vi "Pump Init Selection.vi"(8 "error in (no error)":errorcluster, 11 "Pump Settings In":T1 {"Masterflex"."Pump Number" min=1.0 max=20.0 step=1.0; "Ismatech"."Pump Number" min=1.0 max=20.0 step=1.0; "ASIA Pump C"."channel" min=-1 max=1 step=1}) -> (0 "error out":errorcluster, 2 "Initialized":bool, 3 "Pump Settings Out":T1 {"Masterflex"."Pump Number" min=1.0 max=20.0 step=1.0; "Ismatech"."Pump Number" min=1.0 max=20.0 step=1.0; "ASIA Pump C"."channel" min=-1 max=1 step=1})   [LabVIEW 2018, in "Pump Module.lvlib" / "Pump Module Engine.lvlib"]
uses:
  Pump Module Engine.lvlib
  Pump Settings Cluster.ctl
  Measure Instrument/PID 2 Output Enum.ctl
  Masterflex 7550-30/Controls/Settings Cluster.ctl
  Ismatec ISM 831C/Controls/Ismatech Settings Cluster.ctl
  VICI M50 Party Mode/Settings Cluster.ctl
  Tacmina QI/Tacmina QI DAQ Setting.ctl
  KNF Pump/Settings Cluster plus SIMDOS.ctl
  ASIA Pump/Pump Settings.ctl
  FLOM Pump/Settings Cluster.ctl
  SSI PR Class/SSI PR Settings Cluster.ctl
  Masterflex 75211/Masterflex 75211 DAQ Setting.ctl
  Ismatec ISM 831C/Ismatec ISM 831C.lvlib
  Masterflex 7550-30/Masterflex 7550-30.lvlib
  VICI M50 Party Mode/VICI M6 M50 Party Mode.lvlib
  Tacmina QI/Tacmina QI.lvlib
  KNF Pump/KNF SIMDOS.lvlib
  ASIA Pump.lvlib
  FLOM Pump/FLOM Pump.lvlib
  SSI PR Class/SSI PR Pump.lvlib
  Masterflex 75211/Masterflex 75211.lvlib
  Pump Module.lvlib
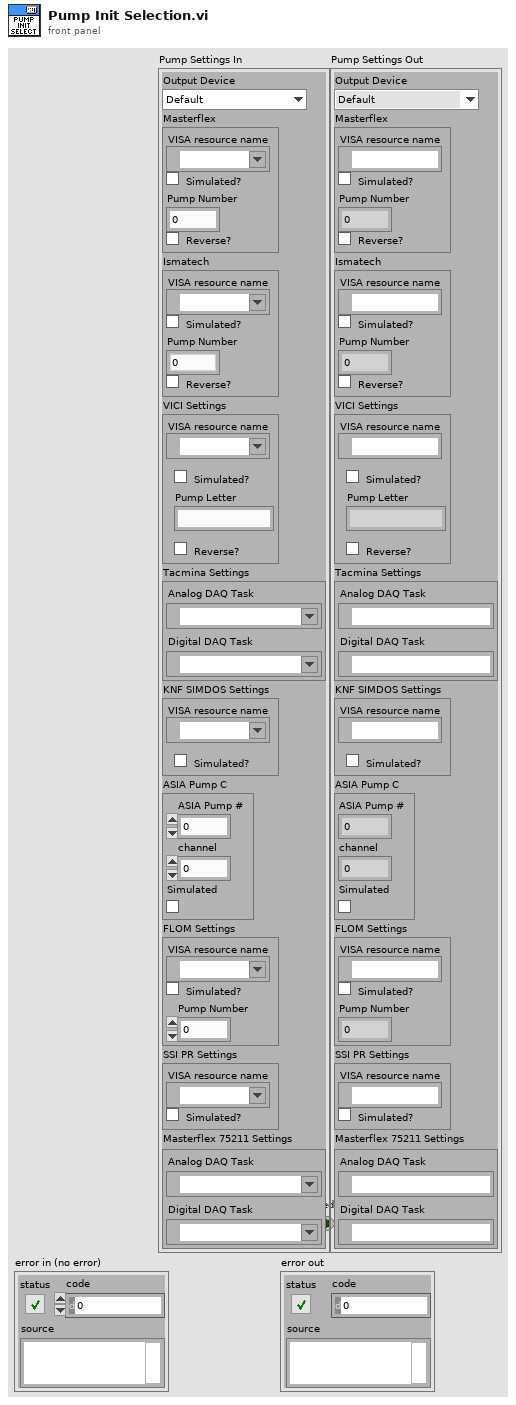
[diagram p1: front panel]
types:
  T1 = typedef "Pump Module.lvlib/Pump Settings Cluster.ctl" = cluster{"Output Device":T2, "Masterflex":T3, "Ismatech":T4, "VICI Settings":T5, "Tacmina Settings":T6, "KNF SIMDOS Settings":T7, "ASIA Pump C":T8, "FLOM Settings":T9, "SSI PR Settings":T10, "Masterflex 75211 Settings":T11}
  T2 = typedef "PID 2 Output Enum.ctl" = enum16{"Default", "Ismatec ISM 831C", "Masterflex 7550-30", "VICI", "Tacmina QI", "KNF SIMDOS", "ASIA Type C", "FLOM UI-22-11", "SSI PR", "Masterflex 75211-70"}
  T3 = typedef "Masterflex 7550-30.lvlib/Settings Cluster.ctl" = cluster{"VISA resource name":refnum<visa-resource-name>, "Simulated?":bool, "Pump Number":dbl, "Reverse?":bool}
  T4 = typedef "Ismatec ISM 831C.lvlib/Ismatech Settings Cluster.ctl" = cluster{"VISA resource name":refnum<visa-resource-name>, "Simulated?":bool, "Pump Number":dbl, "Reverse?":bool}
  T5 = typedef "VICI M6 M50 Party Mode.lvlib/Settings Cluster.ctl" = cluster{"VISA resource name":refnum<visa-resource-name>, "Simulated?":bool, "Pump Letter":string, "Reverse?":bool}
  T6 = typedef "Tacmina QI.lvlib/Tacmina QI DAQ Setting.ctl" = cluster{"Analog DAQ Task":refnum<k21>, "Digital DAQ Task":refnum<k21>}
  T7 = typedef "KNF SIMDOS.lvlib/Settings Cluster plus SIMDOS.ctl" = cluster{"VISA resource name":refnum<visa-resource-name>, "Simulated?":bool}
  T8 = typedef "ASIA Pump.lvlib/Pump Settings.ctl" = cluster{"ASIA Pump #":i32, "channel":i32, "Simulated":bool}
  T9 = typedef "FLOM Pump.lvlib/Settings Cluster.ctl" = cluster{"VISA resource name":refnum<visa-resource-name>, "Simulated?":bool, "Pump Number":dbl}
  T10 = typedef "SSI PR Pump.lvlib/SSI PR Settings Cluster.ctl" = cluster{"VISA resource name":refnum<visa-resource-name>, "Simulated?":bool}
  T11 = typedef "Masterflex 75211.lvlib/Masterflex 75211 DAQ Setting.ctl" = cluster{"Analog DAQ Task":refnum<k21>, "Digital DAQ Task":refnum<k21>}
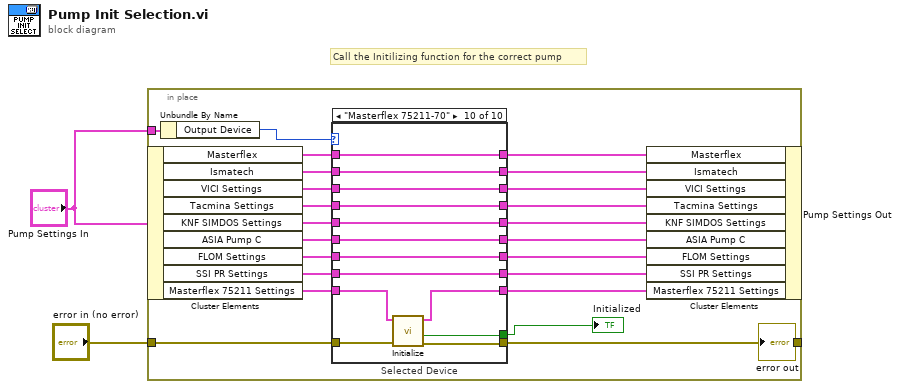
[diagram p0: block diagram]
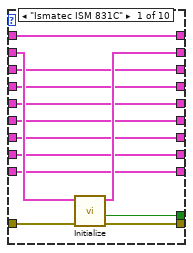
[diagram p2: hidden frame]
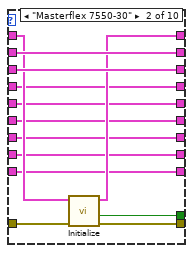
[diagram p3: hidden frame]
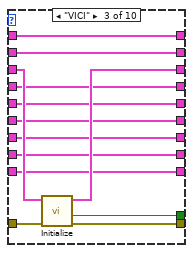
[diagram p4: hidden frame]
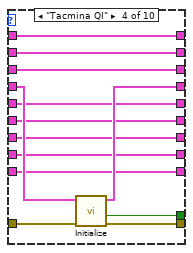
[diagram p5: hidden frame]
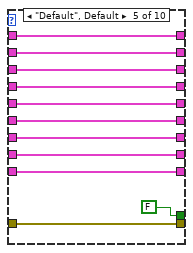
[diagram p6: hidden frame]
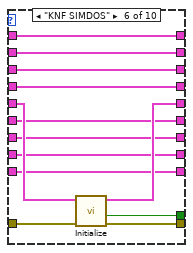
[diagram p7: hidden frame]
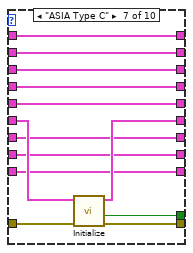
[diagram p8: hidden frame]
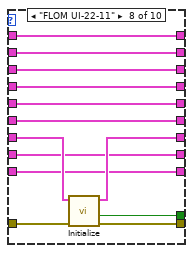
[diagram p9: hidden frame]
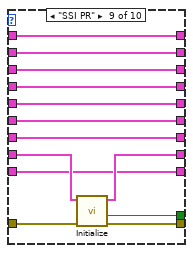
[diagram p10: hidden frame]
diagram:
  # "Call the Initilizing function for the correct pump"
  n1 = in-place {
    in-place-border: [w25] -> w4
    in-place-border: "error in (no error)" -> [w24]
    in-place-border: "Pump Settings In" -> [w23]
    n2 = in-place-cluster #1("Pump Settings In") -> ("Masterflex"=w22:T3, "Ismatech"=w21:T4, "VICI Settings"=w20:T5, "Tacmina Settings"=w19:T6, "KNF SIMDOS Settings"=w18:T7, "ASIA Pump C"=w17:T8, "FLOM Settings"=w16:T9, "SSI PR Settings"=w15:T10, "Masterflex 75211 Settings"=w5:T11)
    n3 = Unbundle By Name(w23) -> ("Output Device"=w26:T2)
    n4 = case "Selected Device" shown="\"Masterflex 75211-70\"" w26 {
      tunnel: w22 -> [w37 w51 w61 w76 w90 w103 w112 w129 w142 w155]
      tunnel: [w37 w50 w61 w76 w90 w103 w112 w129 w142 w155] -> w14
      tunnel: w24 -> [w40 w48 w63 w78 w88 w99 w116 w123 w135 w147]
      tunnel: [w36 w49 w64 w79 w88 w98 w115 w122 w131 w146] -> w25
      tunnel: w21 -> [w39 w53 w62 w77 w89 w102 w111 w128 w141 w154]
      tunnel: [w38 w53 w62 w77 w89 w102 w111 w128 w141 w154] -> w13
      tunnel: w20 -> [w35 w52 w66 w75 w87 w101 w110 w127 w140 w153]
      tunnel: [w35 w52 w65 w75 w87 w101 w110 w127 w140 w153] -> w12
      tunnel: w19 -> [w34 w47 w60 w74 w86 w100 w109 w126 w139 w152]
      tunnel: [w34 w47 w60 w73 w86 w100 w109 w126 w139 w152] -> w11
      tunnel: w18 -> [w33 w46 w59 w72 w85 w96 w108 w125 w138 w151]
      tunnel: [w33 w46 w59 w72 w85 w97 w108 w125 w138 w151] -> w10
      tunnel: [w32 w45 w58 w71 w84 w95 w114 w124 w137 w150] -> w9
      tunnel: w17 -> [w32 w45 w58 w71 w84 w95 w113 w124 w137 w150]
      tunnel: [w31 w44 w57 w70 FALSE ("Initialized") w94 w107 w121 w132 w145] -> w27
      tunnel: [w30 w43 w56 w69 w82 w93 w106 w120 w136 w149] -> w8
      tunnel: w16 -> [w30 w43 w56 w69 w82 w93 w106 w119 w136 w149]
      tunnel: [w29 w42 w55 w68 w81 w92 w105 w118 w133 w148] -> w7
      tunnel: w15 -> [w29 w42 w55 w68 w81 w92 w105 w118 w134 w148]
      tunnel: [w28 w41 w54 w67 w80 w91 w104 w117 w130 w143] -> w6
      tunnel: w5 -> [w28 w41 w54 w67 w80 w91 w104 w117 w130 w144]
      frame "Ismatec ISM 831C" {
        n5 = call "Initialize.vi"("error in (no error)"=w40, "Ismatech Settings"=w39) -> ("error out"=w36:errorcluster, "Initialized"=w31:bool, "Ismatech Settings"=w38:T4)  [unwired: 6 in, 1 out]
      }
      frame "Masterflex 7550-30" {
        n6 = call "Initialize.vi"("error in (no error)"=w48, "Masterflex Settings in"=w51) -> ("error out"=w49:errorcluster, "Initialized"=w44:bool, "Masterflex Settings out"=w50:T3)  [unwired: 6 in, 1 out]
      }
      frame "VICI" {
        n7 = call "Initialize.vi"("error in (no error)"=w63, "VICI Settings"=w66) -> ("error out"=w64:errorcluster, "Initialized"=w57:bool, "VICI Settings"=w65:T5)  [unwired: 6 in, 1 out]
      }
      frame "Tacmina QI" {
        n8 = call "Initialize.vi"("error in"=w78, "Tacmina Settings in"=w74) -> ("error out"=w79:errorcluster, "Initialized"=w70:bool, "Tacmina Settings out"=w73:T6)  [unwired: 7 in]
      }
      frame "Default", Default {
      }
      frame "KNF SIMDOS" {
        n9 = call "Initialize.vi"("error in (no error)"=w99, "KNF Settings In"=w96) -> ("error IO"=w98:errorcluster, "Initialized"=w94:bool, "KNF Settings Out"=w97:T7)  [unwired: 6 in, 1 out]
      }
      frame "ASIA Type C" {
        n10 = call "Initialize.vi"("error in (no error)"=w116, "ASIA Pump C Settings in"=w113) -> ("error out"=w115:errorcluster, "Initialized"=w107:bool, "ASIA Pump C Settings out"=w114:T8)  [unwired: 6 in, 1 out]
      }
      frame "FLOM UI-22-11" {
        n11 = call "Initialize.vi"("error in (no error)"=w123, "FLOM Settings in"=w119) -> ("error out"=w122:errorcluster, "Initialized"=w121:bool, "FLOM Settings out"=w120:T9)  [unwired: 6 in, 1 out]
      }
      frame "SSI PR" {
        n12 = call "Initialize.vi"("error in (no error)"=w135, "SSI PR Settings In"=w134) -> ("error out"=w131:errorcluster, "Initialized"=w132:bool, "SSI PR Settings Out"=w133:T10)  [unwired: 6 in, 1 out]
      }
      frame "Masterflex 75211-70" {
        n13 = call "Initialize.vi"("error in"=w147, "Masterflex 75211 Settings"=w144) -> ("error out"=w146:errorcluster, "Initialized"=w145:bool, "Masterflex 75211 Settings"=w143:T11)  [unwired: 7 in]
      }
    }
    "Initialized" <- w27
    n14 = in-place-cluster #1("Masterflex"=w14, "Ismatech"=w13, "VICI Settings"=w12, "Tacmina Settings"=w11, "KNF SIMDOS Settings"=w10, "ASIA Pump C"=w9, "FLOM Settings"=w8, "SSI PR Settings"=w7, "Masterflex 75211 Settings"=w6) -> (→"Pump Settings Out":T1)
  }
  "error out" <- w4
